vi "Configure Waveform List.vi"(8 "error in (no error)":errorcluster, 10 "Waveform List":string[](array[string]), 11 "VISA resource name":refnum<visa-resource-name>) -> (0 "error out":errorcluster, 3 "VISA resource name out":refnum<visa-resource-name>)   [LabVIEW 2010, in "California Instruments iX Series.lvlib"]
doc: "Configures the waveform sequence list."
uses:
  <instrlib>/California Instruments iX Series/California Instruments iX Series.lvlib
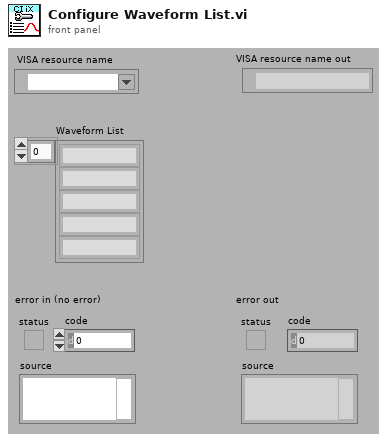
[diagram p1: front panel]
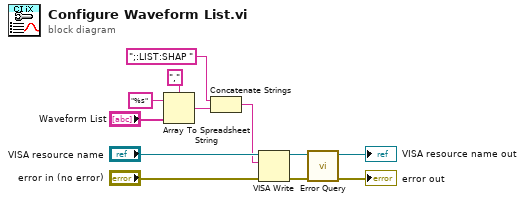
[diagram p0: block diagram]
diagram:
  n1 = Array To Spreadsheet String(delimiter (Tab)=",", array="Waveform List", 3:"%s" ("format string")) -> (spreadsheet string=w3:string)
  n2 = Concatenate Strings(";:LIST:SHAP " ("string"), w3) -> (w1:string)
  n3 = VISA Write(VISA resource name="VISA resource name", write buffer=w1, error in (no error)="error in (no error)") -> (VISA resource name out=w10:refnum<visa-resource-name>, error out=w9:errorcluster)  [unwired: 1 out]
  n4 = call <instrlib>:"Error Query.vi"("error in (no error)"=w9, "VISA resource name"=w10) -> ("error out"=→"error out":errorcluster, "VISA resource name out"=→"VISA resource name out":refnum<visa-resource-name>)  [unwired: 6 in, 2 out]
